vi "Transfer_Curve_2_2400.vi"(0 "File Path":path=path "C:/DATA/raj/transferdump.txt.txt", 1 "V_G Start":dbl=-0.7 format="%#.3g", 3 "V_G Finish":dbl=0.4 format="%#.3g", 4 "V_G Step Size":dbl=0.05 format="%#.3g", 5 "Preread delay (ms)":dbl=10000.0 format="%.2f", 7 "Delay between \naverages (ms)":dbl=200.0 format="%#.3f", 8 "Keithley 237 GPIB address":string="17", 9 "Software Averages":i16=5, 12 "2400":refnum<visa-resource-name>="GPIB0::24::INSTR", 13 "First bias settle (ms)":dbl=60000.0 format="%#.2f", 15 "Current Compliance\nLimit (A) Ke2400":dbl=0.1 format="%#.3e", 18 "Dimensions":T1(ring), 24 "Voltage Compliance Limit 237 (V)":dbl=10.0 format="%#.3f", 25 "Current Compliance\nLimit 237 (A)":dbl=0.1 format="%#.3f", 27 "V_DS":dbl=-0.6 format="%#_13g") -> ()   [LabVIEW 2018]
uses:
  <vilib>/Utility/file.llb/Write Delimited Spreadsheet (string).vi
  Instance           1 16Saved   JV curve .vi
  <instrlib>/Keithley 24XX/Public/Data/Read (Single Point).vi
  <vilib>/Analysis/NI_AALBase.lvlib
  <instrlib>/Keithley 24XX/Keithley 24XX.lvlib
panel:
  in  "2401":refnum<visa-resource-name>="GPIB0::22::INSTR"
  in  "Quick Burn In?":bool
  out "timer":dbl format="%#_6f"
  out "Keithley 2400":cluster{dbl[], dbl[]}(graph)={[-2.0, -1.9, -1.8, -1.7, -1.6, -1.5], [-6.6965744e-11, -6.7804984e-11, -6.685451799999999e-11, -6.6450076e-11, -6.5125542e-11, -6.7339852e-11]}
  out "I_G (A)":dbl=-6.642986e-11 format="%.2e"
  in  "Autozero?":u16(ring) items=["On", "Off", "Once"]
  in  "Measurement Speed (1 PLC)":dbl=1.0 format="%.2g"
  in  "Manual Range (Max I)":dbl=1.0
  in  "Enable Meas Auto Range":bool=TRUE
  in  "Source Mode":u16(ring) items=["Voltage", "Current"]
  in  "Return Sweep?":bool=TRUE
  out "I_DS":dbl=-1.38e-12 format="%.2e"
  out "Outputfile":path=path "C:/DATA/Mark Ziffer/test10"
  in  "Abort Scan":bool=TRUE
  out "V_G":dbl=-1.5 format="%#.2f"
  out "Keithley 237":cluster{dbl[], dbl[]}(graph)={[-2.0, -1.9, -1.8, -1.7, -1.6, -1.5], [-6.720000000000001e-13, -2.18e-13, -2.7599999999999993e-13, -8.999999999999998e-14, -1.3999999999999998e-13, -1.3800000000000002e-13]}
  # "Transfer Curve\nbased on  EL_photocurrent_JV.vi for controlling 2 Ketthleys\n\n9/2017 MZ"
  # "Software Settings"
  # "Ke237 Settings"
  # "Ke2400 Settings"
  # "Notes for IV Scan\n\n2010.07.06 - add absolute value plotter to look at log-scale current\n2010.01.07 - Modified file headers for distinguihing when imported to Igor Pro - the prefix of each header will be the file name.\n2009.01.15 - I updated the code to run on the VISA driver convention. I also modified the file saving and the option to set the\n                      graph display.\n2008.12.01 - I fixed an issue with calculations of J. It was mis-wired to divide current by wavelength, rather than active area.  BM\n\n=========================\nI added the functionality to calculate the fill factor, rectification ratio, short circuit current density, and open circuit voltage. \nAdditionally, current density (mA/cm^2) is reported in the plot window and column B of the data file, and the current (A) has been \nmoved to column C. Open circuit voltage is linearly interpolated. The max power point (mpp) for calculating fill factor is taken as \nthe data point with the highest I-V product, so this makes it only as accurate as your voltage step size, but should be fine for a decent \ndevice on the 50 mV default step size.\n\nIf you know how to use the previous versions of IV scan, \nmake sure you set these parameters before you scan:\n1) Recftification Ratio Bias - this is the +/- bias value you wish to record a rectification ratio at.\n2) Effective Area - this is the area in cm^2 of the diode mask (photoactive area) when measuring under illumination or the measured \n     area of the electrode overlap when measured in dark (regular active area).\n3) Do you want to record a separate data file for the calculated characteristics? If so, make sure the switch is on.\n\nAs of today, I couldn't figure out how to append the computed characteristics to the I-V file without experiencing formating issues, so\nI opted to just create a separate file if you want to save that info. Feel free to fix this if you know how. Check tab 3 > tab 2 > tab 9 in the\nblock diagram.\n\n2008-04-15\nB MacLeod"
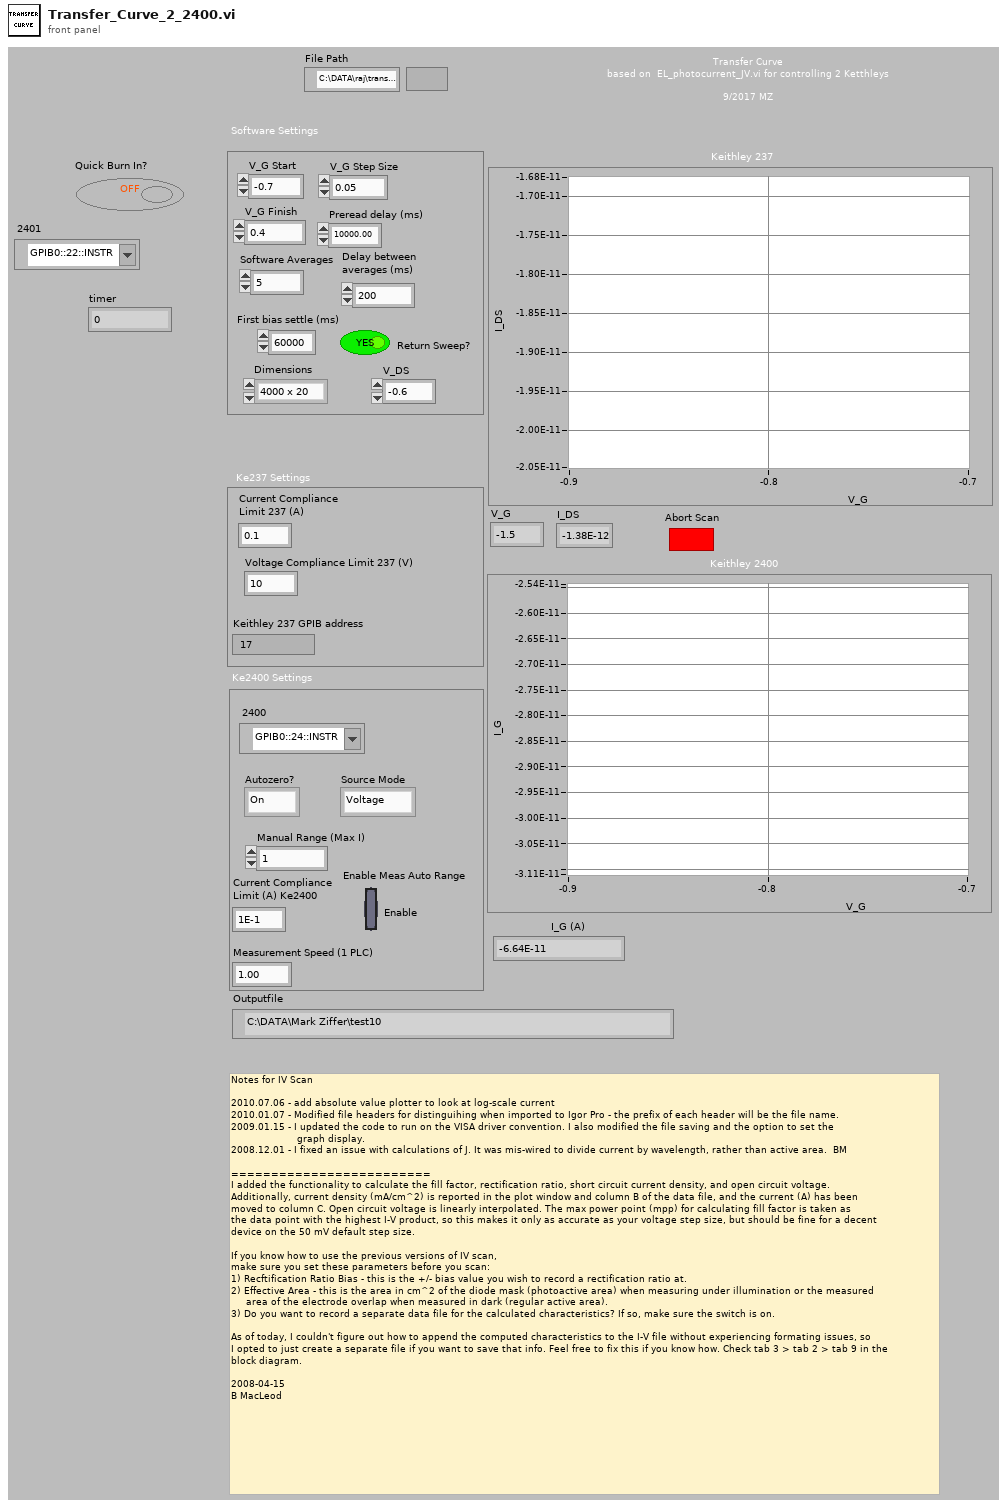
[diagram p1: front panel]
types:
  T1 = enum16{"4000 x 20", "2000 x 20", "1000 x 20", "800 x 20", "400 x 20", "200 x 20", "100 x 20"}
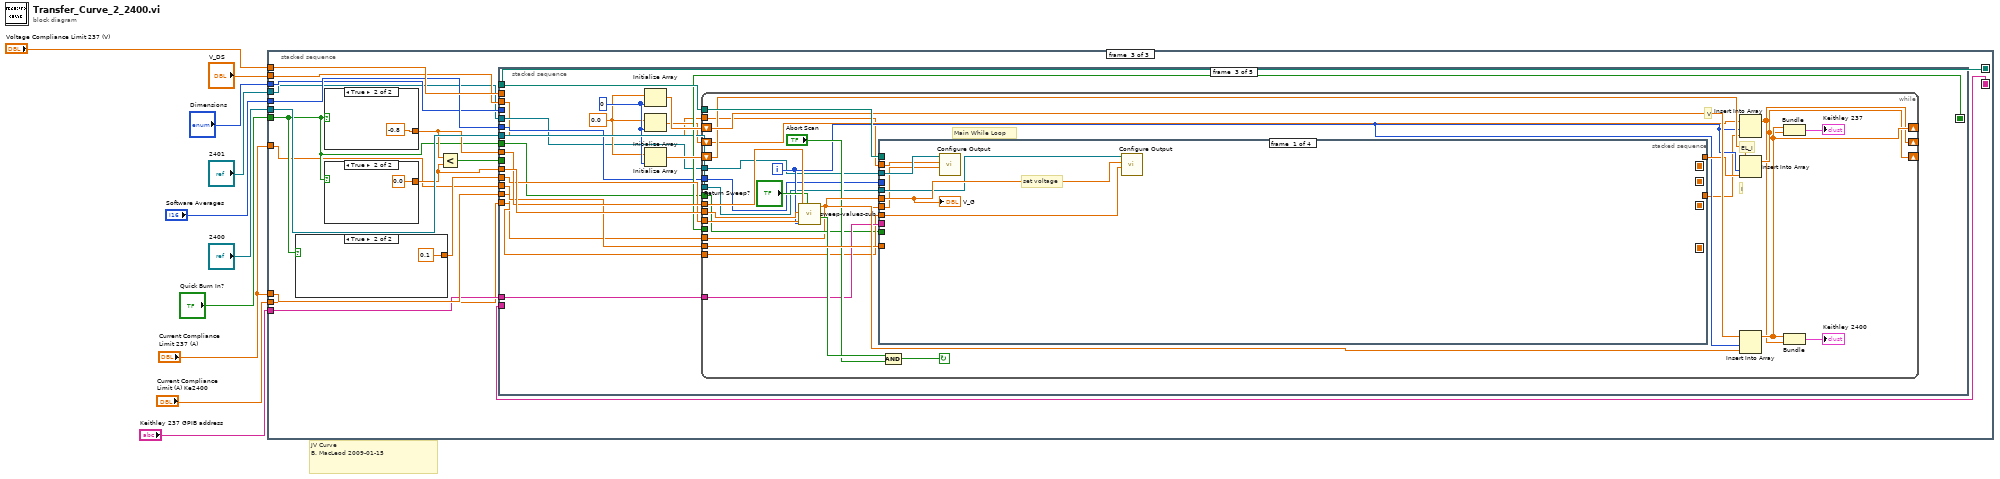
[diagram p0: block diagram]
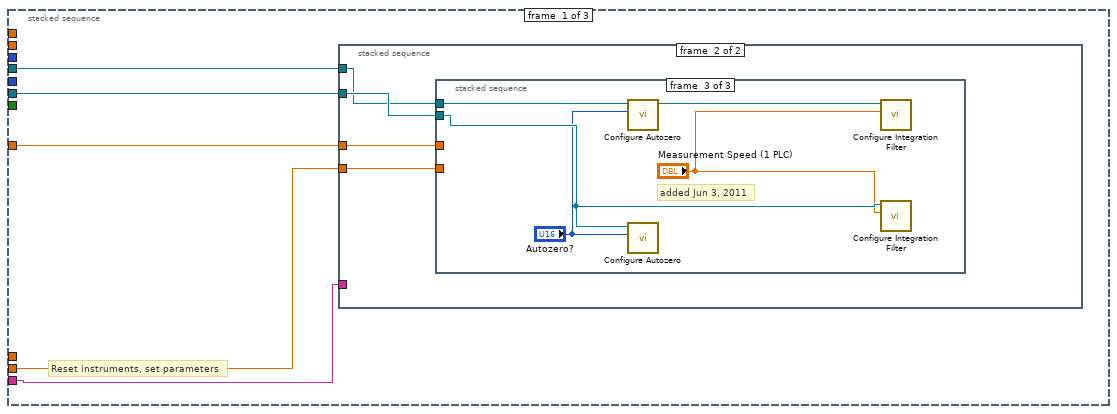
[diagram p2: hidden frame]
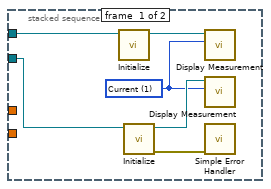
[diagram p3: hidden frame]
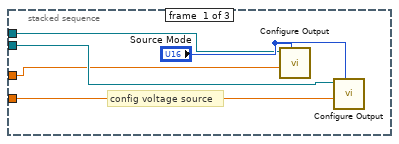
[diagram p4: hidden frame]
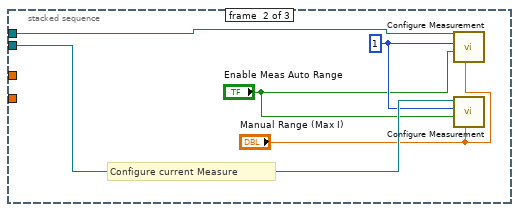
[diagram p5: hidden frame]
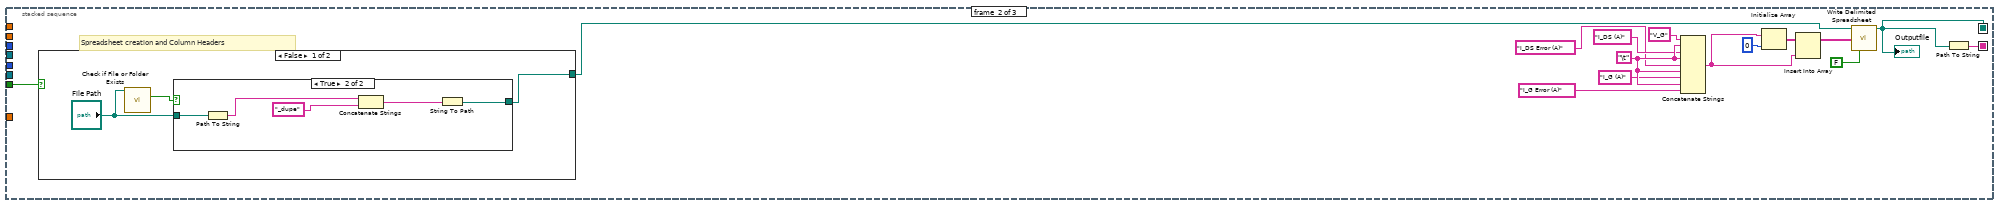
[diagram p6: hidden frame]
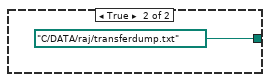
[diagram p8: hidden frame]
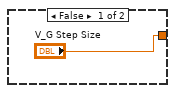
[diagram p9: hidden frame]
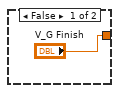
[diagram p10: hidden frame]
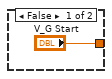
[diagram p11: hidden frame]
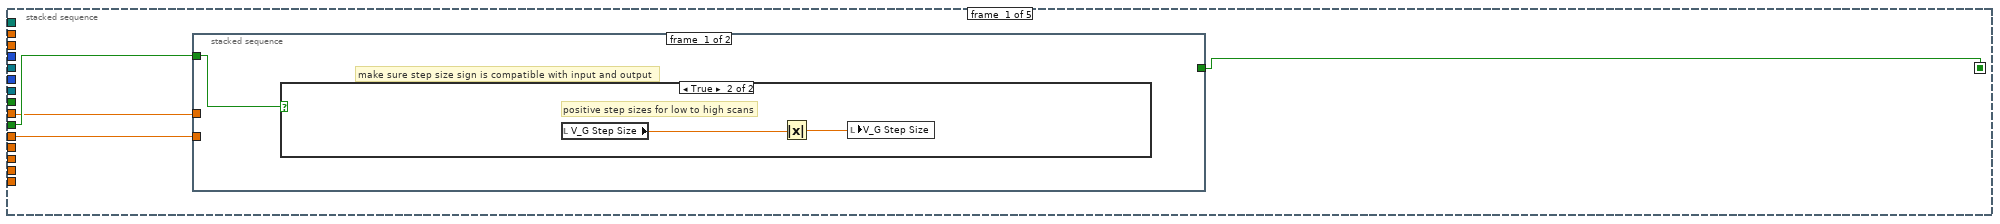
[diagram p12: hidden frame]
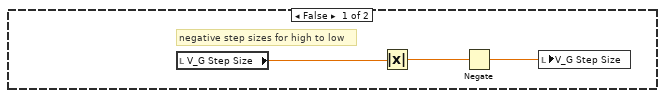
[diagram p13: hidden frame]
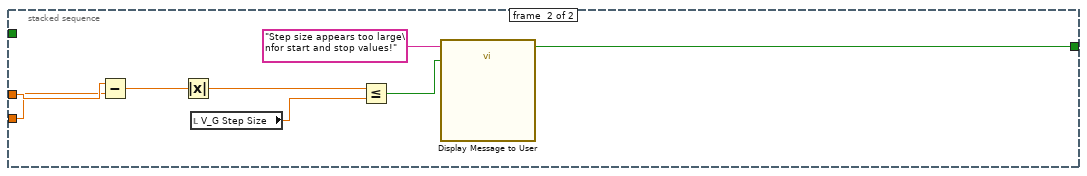
[diagram p14: hidden frame]
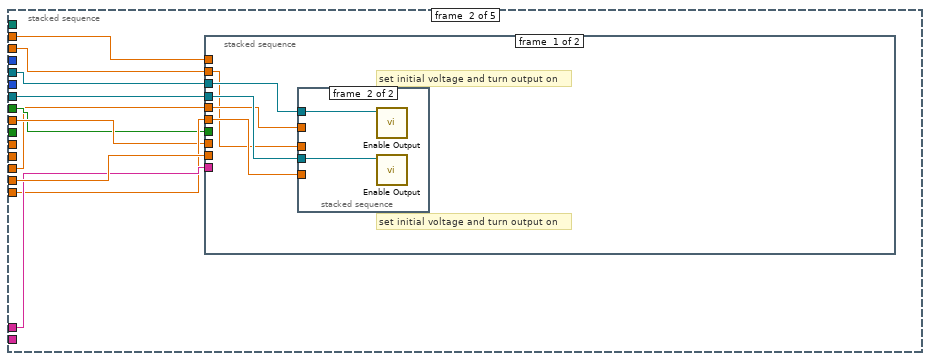
[diagram p15: hidden frame]
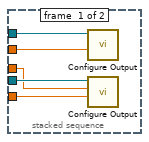
[diagram p16: hidden frame]
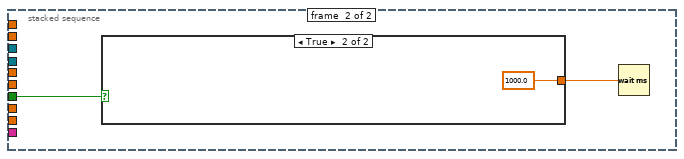
[diagram p17: hidden frame]
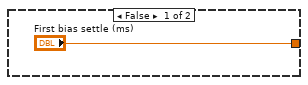
[diagram p18: hidden frame]
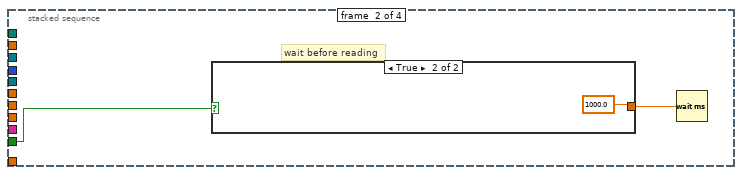
[diagram p19: hidden frame]
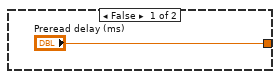
[diagram p20: hidden frame]
diagram:
  # "JV Curve\nB. MacLeod 2009-01-15"
  n1 = stacked-sequence {
    seq-local: [_ w48 _] -> [_ _ w81]
    seq-local: [_ w55 _] -> [_ _ w80]
    tunnel: "Current Compliance\nLimit 237 (A)" -> [_ _ w79]
    tunnel: "Voltage Compliance Limit 237 (V)" -> [_ _ w75]
    tunnel: "Keithley 237 GPIB address" -> [w15 _ w78]
    tunnel: "2400" -> [w14 _ w77]
    tunnel: "Current Compliance\nLimit (A) Ke2400" -> [w13 _ w76]
    tunnel: "V_DS" -> [_ _ w74]
    tunnel: "Software Averages" -> [_ _ w73]
    tunnel: "Dimensions" -> [_ _ w72]
    tunnel: "Quick Burn In?" -> [_ w41 w68]
    tunnel: "2401" -> [w12 _ w67]
    tunnel: "Current Compliance\nLimit 237 (A)" -> [w11 _ w66]
    frame #0 {
      # "Reset instruments, set parameters"
      n2 = stacked-sequence {
        tunnel: w15 -> [_ _]
        tunnel: w14 -> [w21 w25]
        tunnel: w13 -> [_ w24]
        tunnel: w12 -> [w16 w23]
        tunnel: w11 -> [_ w22]
        frame #0 {
          w18 = u16 1 items=["Voltage", "Current", "Resistance"] ("Displayed Measurement (0: Voltage)")
          n3 = call <instrlib>:"Initialize.vi"("VISA resource name"=w16) -> ("VISA resource name out"=w17:refnum<visa-resource-name>)  [unwired: 9 in, 1 out]
          n4 = call <instrlib>:"Initialize.vi"("VISA resource name"=w21) -> ("error out"=w19:errorcluster, "VISA resource name out"=w20:refnum<visa-resource-name>)  [unwired: 9 in]
          n5 = call <instrlib>:"Display Measurement.vi"("Displayed Measurement (0: Voltage)"=w18, "VISA resource name"=w17) -> ()  [unwired: 8 in, 2 out]
          n6 = call <instrlib>:"Display Measurement.vi"("Displayed Measurement (0: Voltage)"=w18, "VISA resource name"=w20) -> ()  [unwired: 8 in, 2 out]
          n7 = call <vilib>:"Simple Error Handler.vi"("error in (no error)"=w19) -> ()  [unwired: 1 in, 8 out]
        }
        frame #1 {
          n8 = stacked-sequence {
            tunnel: w25 -> [w30 w35 w40]
            tunnel: w24 -> [w29 _ _]
            tunnel: w23 -> [w27 w34 w39]
            tunnel: w22 -> [w26 _ _]
            frame #0 {
              # "config voltage source"
              n9 = call <instrlib>:"Configure Output.vi"("Source Mode  (0: Voltage)"="Source Mode", "Compliance  Level (0.1)"=w26, "VISA resource name"=w27) -> ()  [unwired: 3 in, 6 out]
              n10 = call <instrlib>:"Configure Output.vi"("Source Mode  (0: Voltage)"="Source Mode", "Compliance  Level (0.1)"=w29, "VISA resource name"=w30) -> ()  [unwired: 3 in, 6 out]
            }
            frame #1 {
              w32 = 1
              # "Configure current Measure"
              n11 = call <instrlib>:"Configure Measurement.vi"("Manual Range (1.0)"="Manual Range (Max I)", "Enable Auto Range (T:Enable)"="Enable Meas Auto Range", "Function (0: Volts)"=w32, "VISA resource name"=w34) -> ()  [unwired: 1 in, 7 out]
              n12 = call <instrlib>:"Configure Measurement.vi"("Manual Range (1.0)"="Manual Range (Max I)", "Enable Auto Range (T:Enable)"="Enable Meas Auto Range", "Function (0: Volts)"=w32, "VISA resource name"=w35) -> ()  [unwired: 1 in, 7 out]
            }
            frame #2 {
              # "added Jun 3, 2011"
              n13 = call <instrlib>:"Configure Autozero.vi"("Autozero  (0: On)"="Autozero?", "VISA resource name"=w39) -> ("VISA resource name out"=w38:refnum<visa-resource-name>)  [unwired: 1 in, 8 out]
              n14 = call <instrlib>:"Configure Autozero.vi"("Autozero  (0: On)"="Autozero?", "VISA resource name"=w40) -> ()  [unwired: 1 in, 9 out]
              n15 = call <instrlib>:"Configure Integration Filter.vi"("Measurement Speed (1 PLC)"="Measurement Speed (1 PLC)", "VISA resource name"=w38) -> ()  [unwired: 8 in, 2 out]
              n16 = call <instrlib>:"Configure Integration Filter.vi"("Measurement Speed (1 PLC)"="Measurement Speed (1 PLC)", "VISA resource name"=w40) -> ()  [unwired: 8 in, 2 out]
            }
          }
        }
      }
    }
    frame #1 {
      w51 = "\t"
      # "Spreadsheet creation and Column Headers"
      n17 = case shown="False" w41 {
        tunnel: [w56 path "C:/DATA/raj/transferdump.txt"] -> w42
        frame False {
          n18 = call <vilib>:"Check if File or Folder Exists.vi"("path"="File Path") -> ("file or folder exists?"=w58:bool)  [unwired: 8 in, 2 out]
          n19 = case shown="True" w58 {
            tunnel: "File Path" -> [w59 w63]
            tunnel: [w59 w60] -> w56
            frame False {
            }
            frame True {
              n20 = Path To String(path=w63) -> (string=w64:string)
              n21 = Concatenate Strings(w64, "_dupe") -> (w61:string)
              n22 = String To Path(string=w61) -> (path=w60:path)
            }
          }
        }
        frame True {
        }
      }
      n23 = Concatenate Strings("V_G", w51, "I_DS (A)", w51, "I_DS Error (A)", w51, "I_G (A)", w51, "I_G Error (A)" ("string")) -> (w53:string)
      n24 = Initialize Array(w53, 0 ("dimension size")) -> (w52:string[])
      n25 = Insert Into Array(array=w52, new element=w53) -> (w49:string[])  [unwired: 1 in]
      n26 = call-poly <vilib>:"Write Delimited Spreadsheet.vi"("file path (dialog if empty)"=w42, "1D data"=w49, "transpose? (no:F)"=FALSE ("append to file? (new file:F)")) -> ("new file path (Not A Path if cancelled)"=w48:path)  [unwired: 11 in, 1 out]
      "Outputfile" <- w48
      n27 = Path To String(path=w48) -> (string=w55:string)
    }
    frame #2 {
      n28 = case shown="True" w68 {
        tunnel: ["V_G Step Size" 0.1] -> w69
        frame False {
        }
        frame True {
        }
      }
      n29 = case shown="True" w68 {
        tunnel: ["V_G Start" -0.8] -> w71
        frame False {
        }
        frame True {
        }
      }
      n30 = case shown="True" w68 {
        tunnel: ["V_G Finish" 0.0] -> w70
        frame False {
        }
        frame True {
        }
      }
      n31 = Less?(x=w71, y=w70) -> (x < y?=w82:bool)
      n32 = stacked-sequence {
        seq-local: [w89 _ _ _ _] -> [_ _ w144 _ _]
        tunnel: w82 -> [w92 _ _ _ _]
        tunnel: w71 -> [w91 w111 w150 _ _]
        tunnel: w70 -> [w90 _ w151 _ _]
        tunnel: w69 -> [_ _ w149 _ _]
        tunnel: w81 -> [_ _ w148 w232 _]
        tunnel: w80 -> [_ _ _ _ _]
        tunnel: w79 -> [_ w116 w145 _ _]
        tunnel: w78 -> [_ w115 w143 _ w288]
        tunnel: w77 -> [_ w113 w142 _ w287]
        tunnel: w76 -> [_ w114 w138 _ _]
        tunnel: w75 -> [_ w112 _ _ _]
        tunnel: w74 -> [_ w110 w134 w233 _]
        tunnel: w73 -> [_ _ w137 w231 _]
        tunnel: w72 -> [_ _ _ w230 _]
        tunnel: w68 -> [_ w109 w136 _ _]
        tunnel: w67 -> [_ w108 w135 _ _]
        tunnel: w66 -> [_ w107 w133 _ _]
        frame #0 {
          n33 = stacked-sequence {
            tunnel: w92 -> [w93 _]
            tunnel: w91 -> [_ w106]
            tunnel: w90 -> [_ w105]
            tunnel: [_ w99] -> w89
            frame #0 {
              # "make sure step size sign is compatible with input and output"
              n34 = case shown="True" w93 {
                frame False {
                  # "negative step sizes for high to low"
                  n35 = local read "V_G Step Size"() -> (w96:dbl)
                  n36 = Absolute Value(x=w96) -> (abs(x)=w95:dbl)
                  n37 = Negate(x=w95) -> (-x=w94:dbl)
                  n38 = local write "V_G Step Size"(w94) -> ()
                }
                frame True {
                  # "positive step sizes for low to high scans"
                  n39 = local read "V_G Step Size"() -> (w98:dbl)
                  n40 = Absolute Value(x=w98) -> (abs(x)=w97:dbl)
                  n41 = local write "V_G Step Size"(w97) -> ()
                }
              }
            }
            frame #1 {
              n42 = Subtract(x=w106, y=w105) -> (x-y=w104:dbl)
              n43 = Absolute Value(x=w104) -> (abs(x)=w103:dbl)
              n44 = local read "V_G Step Size"() -> (w102:dbl)
              n45 = Less Or Equal?(x=w103, y=w102) -> (x <= y?=w100:bool)
              n46 = call "Display Message to User"("Enable"=w100, "Message"="Step size appears too large\nfor start and stop values!") -> ("OK"=w99:bool)  [unwired: 1 in, 8 out]
            }
          }
        }
        frame #1 {
          n47 = stacked-sequence {
            tunnel: w116 -> [_ _]
            tunnel: w115 -> [_ _]
            tunnel: w114 -> [w121 _]
            tunnel: w113 -> [w120 _]
            tunnel: w112 -> [_ _]
            tunnel: w111 -> [_ _]
            tunnel: w110 -> [w117 _]
            tunnel: w109 -> [_ w130]
            tunnel: w108 -> [w119 _]
            tunnel: w107 -> [w118 _]
            frame #0 {
              # "set initial voltage and turn output on"
              # "set initial voltage and turn output on"
              n48 = stacked-sequence {
                tunnel: w121 -> [w126 _]
                tunnel: w120 -> [w125 w128]
                tunnel: w119 -> [w124 w127]
                tunnel: w118 -> [w123 _]
                tunnel: w117 -> [w122 _]
                frame #0 {
                  n49 = call <instrlib>:"Configure Output.vi"("Compliance  Level (0.1)"=w123, "VISA resource name"=w124) -> ()  [unwired: 4 in, 6 out]
                  n50 = call <instrlib>:"Configure Output.vi"("Compliance  Level (0.1)"=w126, "Output Level (0)"=w122, "VISA resource name"=w125) -> ()  [unwired: 3 in, 6 out]
                }
                frame #1 {
                  n51 = call <instrlib>:"Enable Output.vi"("VISA resource name"=w127) -> ()  [unwired: 2 in, 9 out]
                  n52 = call <instrlib>:"Enable Output.vi"("VISA resource name"=w128) -> ()  [unwired: 2 in, 9 out]
                }
              }
            }
            frame #1 {
              n53 = case shown="True" w130 {
                tunnel: ["First bias settle (ms)" 1000.0] -> w129
                frame False {
                }
                frame True {
                }
              }
              n54 = Wait (ms)(milliseconds to wait=w129) -> ()  [unwired: 1 out]
            }
          }
        }
        frame #2 {
          w141 = 0
          w140 = 0.0
          n55 = Initialize Array(w140, w141) -> (w147:dbl[])
          n56 = Initialize Array(w140, w141) -> (w139:dbl[])
          n57 = Initialize Array(w140, w141) -> (w146:dbl[])
          n58 = while {
            shift-left: w146 -> [w176]
            shift-right: [w164] -> _
            shift-left: w147 -> [w177]
            shift-right: [w167] -> _
            tunnel: w148 -> [w179]
            tunnel: w149 -> [w175]
            tunnel: w150 -> [w174]
            tunnel: w151 -> [w173]
            tunnel: w145 -> [w171]
            tunnel: w144 -> [_]
            shift-right: [w163] -> _
            shift-left: w139 -> [w159]
            tunnel: w143 -> [w162]
            tunnel: w142 -> [w161]
            tunnel: w138 -> [w157]
            tunnel: w137 -> [w156]
            tunnel: w136 -> [w155]
            tunnel: w135 -> [w154]
            tunnel: w134 -> [w153]
            tunnel: w133 -> [w152]
            i -> [w165]
            stop <- w169 continue-if-true
            # "EL_I"
            # "Main While Loop"
            # "V"
            # "I"
            n59 = call "sweep-values-sub.vi"("Forward/Reverse"="Return Sweep?", "Point Number"=w165, "Step Size"=w175, "Sweep Stop"=w173, "Sweep Start"=w174) -> ("Active"=w170:bool, "Output"=w178:dbl)  [unwired: 2 out]
            n60 = stacked-sequence {
              seq-local: [_ _ w200 _] -> [_ _ _ w214]
              seq-local: [_ _ w195 _] -> [_ _ _ w215]
              seq-local: [_ _ w197 _] -> [_ _ _ w213]
              seq-local: [_ _ w196 _] -> [_ _ _ w212]
              tunnel: [_ _ w195 _] -> w166
              tunnel: w178 -> [w186 _ _ w226]
              tunnel: w179 -> [_ _ _ w217]
              tunnel: w171 -> [_ _ _ _]
              tunnel: w162 -> [_ _ w199 _]
              tunnel: w161 -> [w184 _ w198 _]
              tunnel: [_ _ w197 _] -> w160
              tunnel: w157 -> [w185 _ _ _]
              tunnel: w156 -> [_ _ w194 _]
              tunnel: w155 -> [_ w187 _ _]
              tunnel: w154 -> [w183 _ w192 _]
              tunnel: w153 -> [w182 _ _ _]
              tunnel: w152 -> [w181 _ _ _]
              frame #0 {
                # "set voltage"
                n61 = call <instrlib>:"Configure Output.vi"("Compliance  Level (0.1)"=w181, "Output Level (0)"=w182, "VISA resource name"=w183) -> ()  [unwired: 3 in, 6 out]
                n62 = call <instrlib>:"Configure Output.vi"("Compliance  Level (0.1)"=w185, "Output Level (0)"=w186, "VISA resource name"=w184) -> ()  [unwired: 3 in, 6 out]
                "V_G" <- w186
              }
              frame #1 {
                # "wait before reading"
                n63 = case shown="True" w187 {
                  tunnel: ["Preread delay (ms)" 1000.0] -> w188
                  frame False {
                  }
                  frame True {
                  }
                }
                n64 = Wait (ms)(milliseconds to wait=w188) -> ()  [unwired: 1 out]
              }
              frame #2 {
                # "I_DS"
                # "I_G"
                # "read values"
                n65 = for {
                  N: w194 -> [_]
                  tunnel: w199 -> [w205]
                  tunnel: w198 -> [w204]
                  tunnel: [w203] -> w193 mode=indexing
                  tunnel: w192 -> [w202]
                  tunnel: [w201] -> w191 mode=indexing
                  n66 = stacked-sequence {
                    tunnel: w205 -> [_ _]
                    tunnel: w204 -> [w209 _]
                    tunnel: [w208 _] -> w203
                    tunnel: w202 -> [w207 _]
                    tunnel: [w206 _] -> w201
                    frame #0 {
                      n67 = call-poly <instrlib>:"Read.vi"("VISA resource name"=w207) -> ("Current"=w206:sgl)  [unwired: 8 in, 6 out]
                      "I_DS" <- w206
                      n68 = call-poly <instrlib>:"Read.vi"("VISA resource name"=w209) -> ("Current"=w208:sgl)  [unwired: 8 in, 6 out]
                      "I_G (A)" <- w208
                    }
                    frame #1 {
                      n69 = Wait (ms)(milliseconds to wait="Delay between \naverages (ms)") -> (millisecond timer value=→"timer":u32)
                    }
                  }
                }
                n70 = call <vilib>:"Std Deviation and Variance.vi"("X"=w193) -> ("mean"=w197:dbl, "standard deviation"=w196:dbl)  [unwired: 1 in, 1 out]
                n71 = call <vilib>:"Std Deviation and Variance.vi"("X"=w191) -> ("mean"=w195:dbl, "standard deviation"=w200:dbl)  [unwired: 1 in, 1 out]
              }
              frame #3 {
                w221 = "\t"
                # "I_G"
                # "write data to file"
                # "X"
                n72 = Format Into String(format string="%#f", w226) -> (resulting string=w224:string)  [unwired: 2 in, 1 out]
                n73 = Number To Exponential String(number=w215) -> (E-format string=w227:string)  [unwired: 3 out]
                n74 = Number To Exponential String(number=w214) -> (E-format string=w223:string)  [unwired: 3 out]
                n75 = Number To Exponential String(number=w212) -> (E-format string=w219:string)  [unwired: 3 out]
                n76 = Number To Exponential String(number=w213) -> (E-format string=w220:string)  [unwired: 3 out]
                n77 = Concatenate Strings(w224, w221, w227, w221, w223, w221, w220, w221, w219) -> (w222:string)
                n78 = Build Array(w222) -> (w218:string[])
                n79 = call-poly <vilib>:"Write Delimited Spreadsheet.vi"("file path (dialog if empty)"=w217, "1D data"=w218, "append to file? (new file:F)"=TRUE) -> ()  [unwired: 11 in, 2 out]
              }
            }
            n80 = Compound Arithmetic op=AND(w170, "Abort Scan") -> (w169:bool)
            n81 = Insert Into Array(array=w159, index=w165, new element=w160) -> (w163:dbl[])
            n82 = Insert Into Array(array=w176, index=w165, new element=w166) -> (w164:dbl[])
            n83 = Insert Into Array(array=w177, index=w165, new element=w178) -> (w167:dbl[])
            n84 = Bundle(w167, w164) -> (→"Keithley 237":cluster{dbl[], dbl[]})  [unwired: 1 out]
            n85 = Bundle(w167, w163) -> (→"Keithley 2400":cluster{dbl[], dbl[]})  [unwired: 1 out]
          }
        }
        frame #3 {
          n86 = case shown="\"2000 x 20\"" w230 {
            tunnel: [4000 2000 1000 800 400 200 100] -> w229
            tunnel: [20 20 20 20 20 20 20] -> w228
            frame "4000 x 20", Default {
            }
            frame "2000 x 20" {
            }
            frame "1000 x 20" {
            }
            frame "800 x 20" {
            }
            frame "400 x 20" {
            }
            frame "200 x 20" {
            }
            frame "100 x 20" {
            }
          }
          n87 = stacked-sequence {
            tunnel: w233 -> [_ w259 _ _ _]
            tunnel: w232 -> [w248 w257 w263 w278 w280]
            tunnel: w231 -> [_ _ w265 _ _]
            tunnel: w229 -> [_ _ _ w273 _]
            tunnel: w228 -> [_ _ _ _ w279]
            frame #0 {
              w253 = ""
              w252 = "\t"
              n88 = Concatenate Strings(w253, w252, w253, w252) -> (w249:string)
              n89 = Build Array(w249) -> (w251:string[])
              n90 = call-poly <vilib>:"Write Delimited Spreadsheet.vi"("file path (dialog if empty)"=w248, "1D data"=w251, "append to file? (new file:F)"=TRUE) -> ()  [unwired: 11 in, 2 out]
            }
            frame #1 {
              w260 = "\t"
              n91 = Number To Fractional String(number=w259, precision (6)=3) -> (F-format string=w258:string)  [unwired: 2 in]
              n92 = Concatenate Strings("V_DS = ", w260, w258, w260) -> (w261:string)
              n93 = Build Array(w261) -> (w256:string[])
              n94 = call-poly <vilib>:"Write Delimited Spreadsheet.vi"("file path (dialog if empty)"=w257, "1D data"=w256, "append to file? (new file:F)"=TRUE) -> ()  [unwired: 11 in, 2 out]
            }
            frame #2 {
              w268 = "\t"
              n95 = Number To Decimal String(number=w265) -> (decimal integer string=w264:string)  [unwired: 1 in]
              n96 = Concatenate Strings("Number of Averages = ", w268, w264, w268) -> (w269:string)
              n97 = Build Array(w269) -> (w267:string[])
              n98 = call-poly <vilib>:"Write Delimited Spreadsheet.vi"("file path (dialog if empty)"=w263, "1D data"=w267, "append to file? (new file:F)"=TRUE) -> ()  [unwired: 11 in, 2 out]
            }
            frame #3 {
              w275 = "\t"
              n99 = Number To Decimal String(number=w273) -> (decimal integer string=w274:string)  [unwired: 1 in]
              n100 = Concatenate Strings("Width/um =", w275, w274, w275) -> (w272:string)
              n101 = Build Array(w272) -> (w271:string[])
              n102 = call-poly <vilib>:"Write Delimited Spreadsheet.vi"("file path (dialog if empty)"=w278, "1D data"=w271, "append to file? (new file:F)"=TRUE) -> ()  [unwired: 11 in, 2 out]
            }
            frame #4 {
              w281 = "\t"
              n103 = Number To Decimal String(number=w279) -> (decimal integer string=w284:string)  [unwired: 1 in]
              n104 = Concatenate Strings("Length/um =", w281, w284, w281) -> (w285:string)
              n105 = Build Array(w285) -> (w286:string[])
              n106 = call-poly <vilib>:"Write Delimited Spreadsheet.vi"("file path (dialog if empty)"=w280, "1D data"=w286, "append to file? (new file:F)"=TRUE) -> ()  [unwired: 11 in, 2 out]
            }
          }
        }
        frame #4 {
          # "reset instrument at end of sweep"
          n107 = call <instrlib>:"Reset.vi"("VISA resource name"=w287) -> ()  [unwired: 9 in, 2 out]
          n108 = call <userlib>:"Keith 237 Reset.vi"("GPIB address"=w288) -> ()  [unwired: 1 in, 1 out]
        }
      }
    }
  }
